vi "Get TDC Measurement.vi"(8 "error in":errorcluster, 11 "FPGA VI Reference In":T1) -> (0 "error out":errorcluster, 1 "tdc ever rollover":bool, 2 "tdc measurement":u16, 3 "FPGA VI Reference Out":T1, 4 "Timed Out?":bool, 5 "measurement is valid after arm":bool)   [LabVIEW 2011, in "FlexRIO Host Library (User).lvlib"]
uses:
  FlexRIO Host Library (User).lvlib
  Session/FPGA Session Ref.ctl
  <vilib>/rvi/interface/nirviReadWriteControl/nirviReadWriteControl.xnode
  Zeiss Acquisition Demo/FPGA Bitfiles/FlexRIODigitizer_FPGABoard_Acquire_Rev2.lvbitx
  <vilib>/rvi/errors/niLvFpgaMergeErrorWithErrorCode.vi
  <vilib>/rvi/errors/niLvFpgaAdjustHostInterfaceError.vi
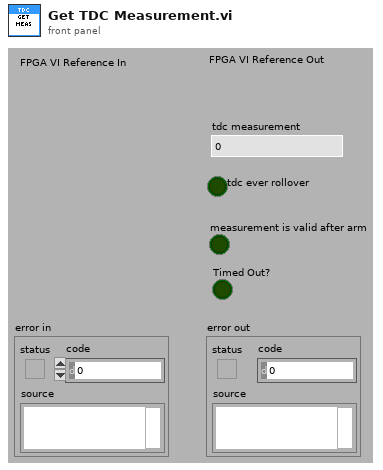
[diagram p1: front panel]
types:
  T1 = typedef "FlexRIO Host.lvlib/FPGA Session Ref.ctl" = refnum<k20>
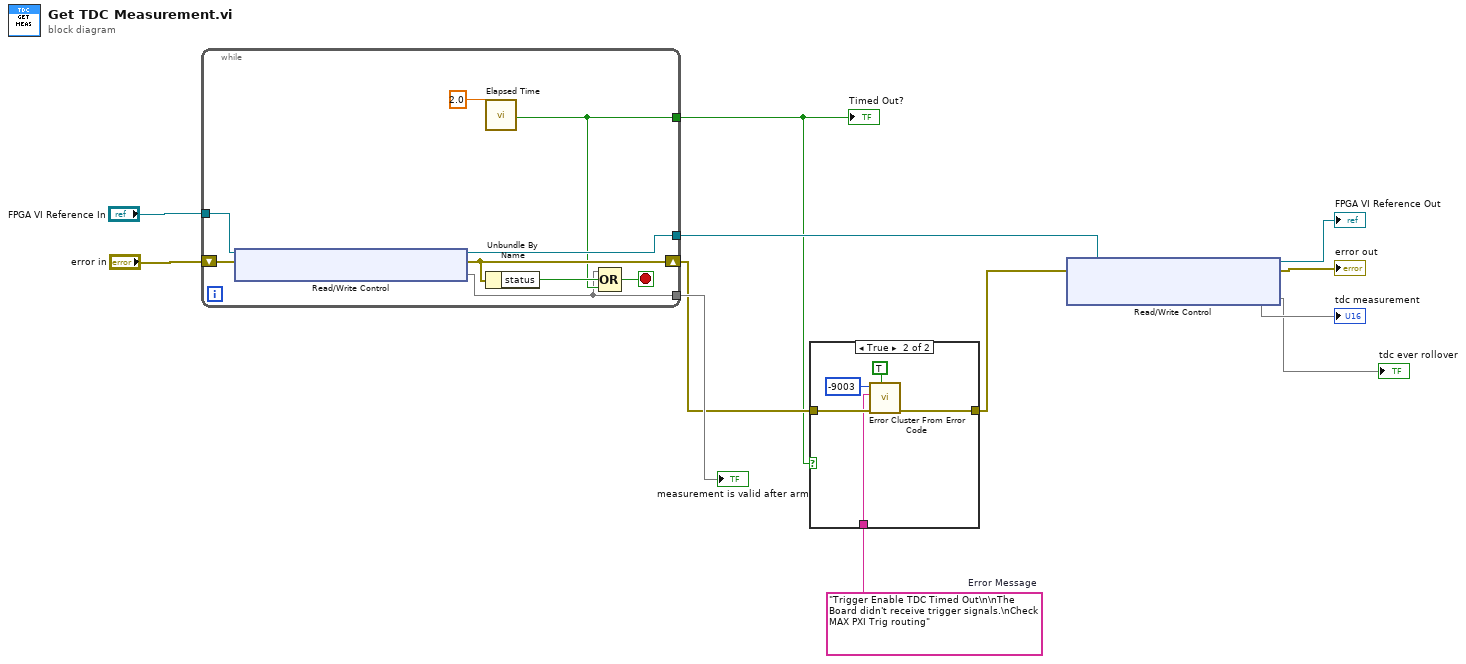
[diagram p0: block diagram]
diagram:
  w5 = "Trigger Enable TDC Timed Out\n\nThe Board didn't receive trigger signals.\nCheck MAX PXI Trig routing"  # Error Message
  n1 = while {
    tunnel: [w20] -> w9
    tunnel: "FPGA VI Reference In" -> [w18]
    shift-right: [w21] -> w3
    shift-left: "error in" -> [w19]
    tunnel: [w15] -> w2
    tunnel: [w14] -> w6
    stop <- w16 stop-if-true
    n2 = xnode "Read/Write Control"("FPGA VI Reference In"=w18, "error in"=w19) -> ("FPGA VI Reference Out"=w20:T1, "error out"=w21:errorcluster, "TDC Measurement.measurement is valid"=w14)
    n3 = call "Elapsed Time"("Time Target (s)"=2.0) -> ("Time has Elapsed"=w15:bool)  [unwired: 11 in, 7 out]
    n4 = Unbundle By Name(w21) -> ("status"=w17:bool)
    n5 = Compound Arithmetic op=OR(w14, w17, w15) -> (w16:bool)
  }
  "Timed Out?" <- w2
  "measurement is valid after arm" <- w6
  n6 = case shown="True" w2 {
    tunnel: w3 -> [w22 w26]
    tunnel: [w22 w25] -> w4
    tunnel: w5 -> [_ w24]
    frame False {
    }
    frame True {
      n7 = call <vilib>:"Error Cluster From Error Code.vi"("show call chain? (False)"=TRUE, "error in (no error)"=w26, "error message (\"\")"=w24, "error code (0)"=-9003) -> ("error out"=w25:errorcluster)  [unwired: 5 in]
    }
  }
  n8 = xnode "Read/Write Control"("FPGA VI Reference In"=w9, "error in"=w4) -> ("FPGA VI Reference Out"=→"FPGA VI Reference Out":T1, "error out"=→"error out":errorcluster, "TDC Measurement.tdc measurement"=→"tdc measurement", "TDC Measurement.tdc ever rollover"=→"tdc ever rollover")
